vi "UserInterfaceEventPattern 3.vi"() -> ()   [LabVIEW 2014]
doc: "이 템플릿을 사용하여 사용자 인터페이스 이벤트 핸들러 디자인 패턴을 생성합니다. 대화 상자 및 다른 사용자 인터페이스에 대하여 이 패턴을 사용합니다. 또한, VI가 사용자 인터페이스 이벤트를 같은 방법으로 다룰 수 있는, 사용자 정의 이벤트를 생성하고 실행할 수 있습니다."
panel:
  in  "Button 1":bool caption="버튼 1"
  in  "stop":bool caption="정지"
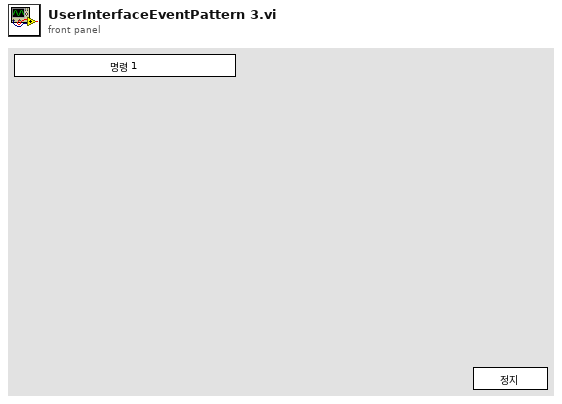
[diagram p1: front panel]
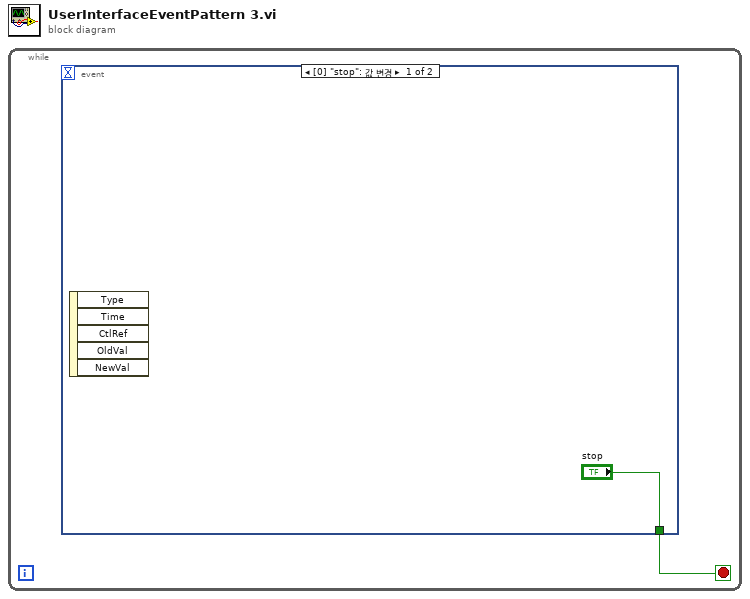
[diagram p0: block diagram]
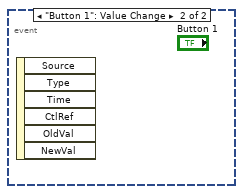
[diagram p2: hidden frame]
diagram:
  n1 = while {
    stop <- w1 stop-if-true
    n2 = event shown="[0] \"stop\": 값 변경" {
      selector: _ -> [_ _]
      dyn-events: _ -> [_ _]
      timeout: _ -> [_ _]
      tunnel: ["stop" _] -> w1
      event "stop": Value Change {
        n3 = event-data() -> ()  [unwired: 1 in, 5 out]
      }
      event "Button 1": Value Change {
        n4 = event-data() -> ()  [unwired: 1 in, 6 out]
      }
    }
  }
